vi "1A_Thermistor_Offset_Calibrations.vi"(7 "Offset Ratio":dbl format="%_6g", 8 "Ideal Abort Threshold (R @ 42C)":dbl=46875.0, 9 "Ideal Critical Threshold (R @ 41C)":dbl=48917.0, 10 "Ideal Warning Threshold (R @ 40C)":dbl=51060.0, 11 "Ideal Minimum Threshold (R @ 10C)":dbl=207801.0) -> (0 "Cal Abort Threshold (R/4)":u16, 1 "Cal Critical Threshold (R/4)":u16, 2 "Cal Warning Threshold (R/4)":u16, 3 "Cal Minimum Threshold (R/4)":u16)   [LabVIEW 2010]
doc: "Temperature offsets are calculated using the SP21629 thermistor spline interpolation function."
panel:
  out "Temp Offset Abort":dbl
  out "Temp Offset Critical":dbl
  out "Temp Offset Warning":dbl
  out "Temp Offset Minimum":dbl
  out "Adjusted Abort Threshold (R)":dbl
  out "Adjusted Critical Threshold (R)":dbl
  out "Adjusted Warning Threshold (R)":dbl
  out "Adjusted Minimum Threshold (R)":dbl
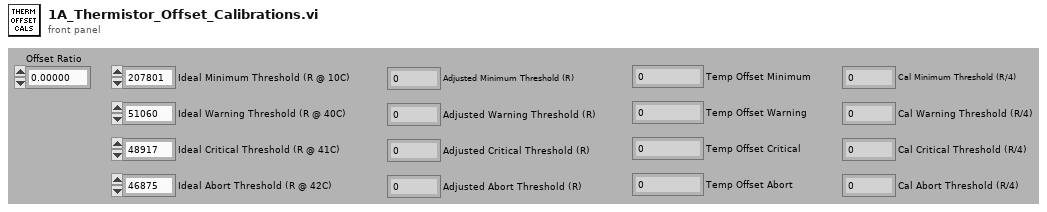
[diagram p1: front panel]
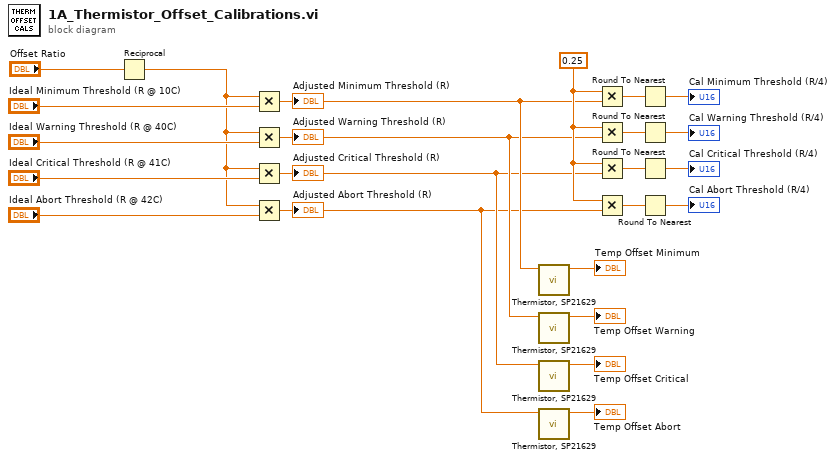
[diagram p0: block diagram]
diagram:
  w14 = 0.25 ("x")
  n1 = Reciprocal(x="Offset Ratio") -> (1/x=w1:dbl)
  n2 = Multiply(x=w1, y="Ideal Minimum Threshold (R @ 10C)") -> (x*y=w7:dbl)
  "Adjusted Minimum Threshold (R)" <- w7
  n3 = Multiply(x=w1, y="Ideal Warning Threshold (R @ 40C)") -> (x*y=w6:dbl)
  "Adjusted Warning Threshold (R)" <- w6
  n4 = Multiply(x=w1, y="Ideal Critical Threshold (R @ 41C)") -> (x*y=w5:dbl)
  "Adjusted Critical Threshold (R)" <- w5
  n5 = Multiply(x=w1, y="Ideal Abort Threshold (R @ 42C)") -> (x*y=w4:dbl)
  "Adjusted Abort Threshold (R)" <- w4
  n6 = call "Thermistor, SP21629.vi"("resistance (ohms)"=w7) -> ("temperature (C)"=→"Temp Offset Minimum":dbl)  [unwired: 9 in, 1 out]
  n7 = call "Thermistor, SP21629.vi"("resistance (ohms)"=w6) -> ("temperature (C)"=→"Temp Offset Warning":dbl)  [unwired: 9 in, 1 out]
  n8 = call "Thermistor, SP21629.vi"("resistance (ohms)"=w5) -> ("temperature (C)"=→"Temp Offset Critical":dbl)  [unwired: 9 in, 1 out]
  n9 = call "Thermistor, SP21629.vi"("resistance (ohms)"=w4) -> ("temperature (C)"=→"Temp Offset Abort":dbl)  [unwired: 9 in, 1 out]
  n10 = Multiply(x=w14, y=w7) -> (x*y=w13:dbl)
  n11 = Multiply(x=w14, y=w6) -> (x*y=w12:dbl)
  n12 = Multiply(x=w14, y=w5) -> (x*y=w11:dbl)
  n13 = Multiply(x=w14, y=w4) -> (x*y=w10:dbl)
  n14 = Round To Nearest(number=w13) -> (nearest integer value=→"Cal Minimum Threshold (R/4)":dbl)
  n15 = Round To Nearest(number=w12) -> (nearest integer value=→"Cal Warning Threshold (R/4)":dbl)
  n16 = Round To Nearest(number=w11) -> (nearest integer value=→"Cal Critical Threshold (R/4)":dbl)
  n17 = Round To Nearest(number=w10) -> (nearest integer value=→"Cal Abort Threshold (R/4)":dbl)
